vi "Send Tree Item Open.vi"(5 "EventFilter Reference":T1, 8 "Item Tag":string, 9 "Time":u32, 10 "CtlRef":refnum<vi>, 11 "Message Enqueuer in":refnum<class "Message Enqueuer.lvclass">) -> (0 "error out":errorcluster, 3 "Filtered EventDataMessage":refnum<class "TreeItemOpenMsg.lvclass">)   [LabVIEW 2020, in "MVA Framework.lvlib" / "ActorEvents.lvlib" / "TreeItemOpenMsg.lvclass"]
doc: "发送树形项打开事件消息"
uses:
  TreeItemOpenMsg.lvclass
  <vilib>/ActorFramework/Message Enqueuer/Message Enqueuer.lvclass
  IEventFilter/EventFilter Reference.ctl
  IEventFilter/IEventFilter.lvclass
  TreeItemOpenMsg.lvclass/TreeItemOpenMsg.ctl
  EventDataMessage/EventDataMessage.lvclass/EventDataMessage.ctl
  <vilib>/ActorFramework/Message Enqueuer/Message Enqueuer.lvclass/Message Enqueuer.ctl
  <vilib>/ActorFramework/Message Enqueuer/Enqueue.vi
  <vilib>/Utility/error.llb/Clear Errors.vi
  EventDataMessage/EventDataMessage.lvclass
  C:/Program Files/National Instruments/LabVIEW 2020/vi.lib/ActorFramework/Message/Message.lvclass
  <vilib>/ActorFramework/Message Priority Queue/Priority Enqueue.vi
panel:
  in  "error in (no error)":errorcluster
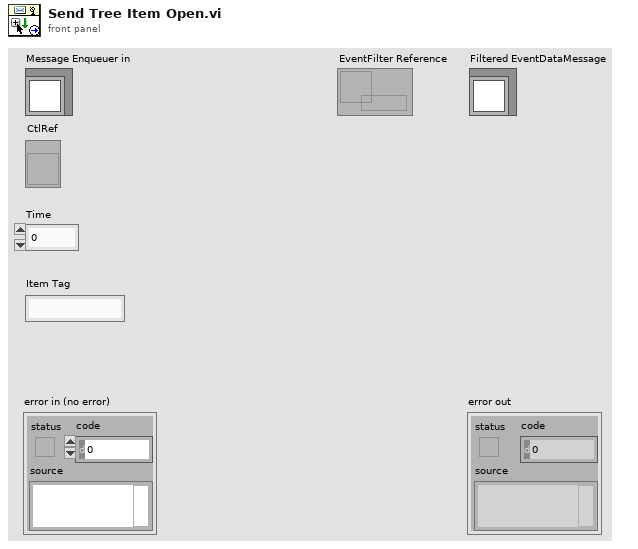
[diagram p1: front panel]
types:
  T1 = typedef "MVA Framework.lvlib/ActorEvents.lvlib/IEventFilter.lvclass/EventFilter Reference.ctl" = refnum<data-value>
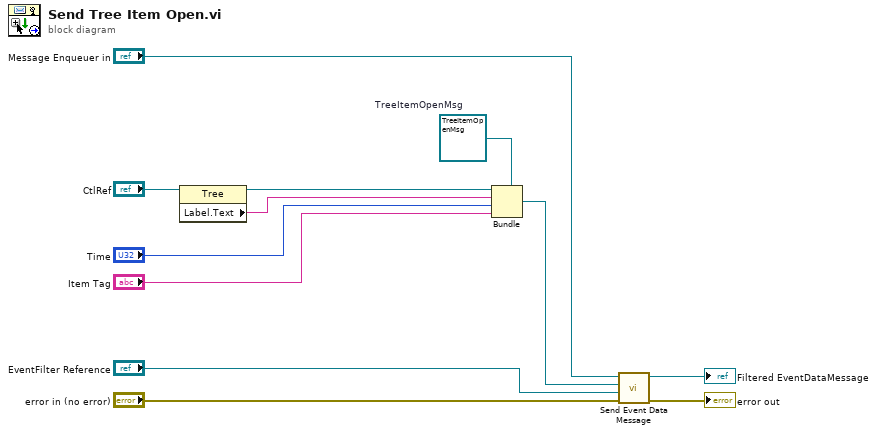
[diagram p0: block diagram]
diagram:
  w12 = refnum<class "TreeItemOpenMsg.lvclass"> refnum  # TreeItemOpenMsg
  n1 = property class="Tree"(reference="CtlRef") -> (reference out=w4:refnum<vi>, "Label.Text"=w6:string)  [unwired: 1 in, 1 out]
  n2 = Bundle(cluster=w12, w4, w6, "Time", "Item Tag") -> (w9:refnum<class "TreeItemOpenMsg.lvclass">)
  n3 = call "Send Event Data Message.vi"("error in (no error)"="error in (no error)", "EventFilter Reference"="EventFilter Reference", "EventDataMessage"=w9, "Message Enqueuer in"="Message Enqueuer in") -> ("error out"=→"error out":errorcluster, "Filtered EventDataMessage"=→"Filtered EventDataMessage":refnum<class "TreeItemOpenMsg.lvclass">)  [unwired: 6 in]
